vi "SignalObservation_NB.vi"(6 "error in (no error)":errorcluster, 8 "PllCharz Divider":string(combo)="Div1", 9 "Signal":string(combo)="VCO") -> (0 "error out":errorcluster)   [LabVIEW 2011]
doc: "This VI outputs a selected signal from the NB PLL.\n\nInputs:\n1. Signal: PLL Clock to output (Refclk, VCO, etc.).\n2. PllCharz Divider: Setting of the PllCharz divider (Div1 or Div16)."
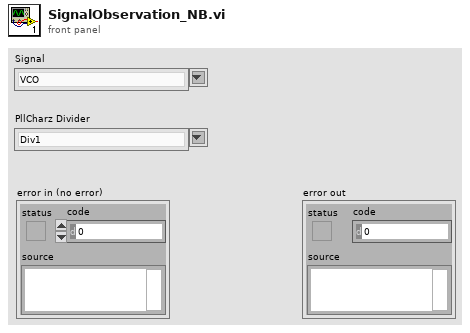
[diagram p1: front panel]
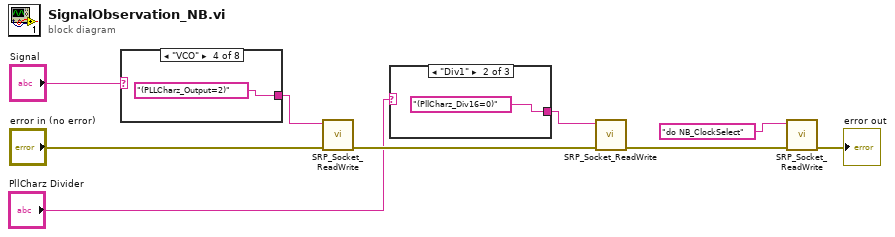
[diagram p0: block diagram]
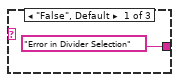
[diagram p2: hidden frame]
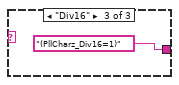
[diagram p3: hidden frame]
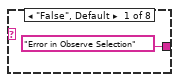
[diagram p4: hidden frame]
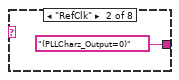
[diagram p5: hidden frame]
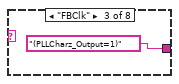
[diagram p6: hidden frame]
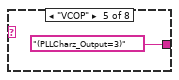
[diagram p7: hidden frame]
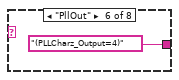
[diagram p8: hidden frame]
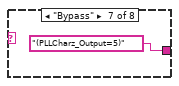
[diagram p9: hidden frame]
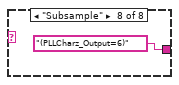
[diagram p10: hidden frame]
diagram:
  n1 = case shown="\"VCO\"" "Signal" {
    tunnel: ["Error in Observe Selection" "(PLLCharz_Output=0)" "(PLLCharz_Output=1)" "(PLLCharz_Output=2)" "(PLLCharz_Output=3)" "(PLLCharz_Output=4)" "(PLLCharz_Output=5)" "(PLLCharz_Output=6)"] -> w5
    frame "False", Default {
    }
    frame "RefClk" {
    }
    frame "FBClk" {
    }
    frame "VCO" {
    }
    frame "VCOP" {
    }
    frame "PllOut" {
    }
    frame "Bypass" {
    }
    frame "Subsample" {
    }
  }
  n2 = call "SRP_Socket_ReadWrite.vi"("error in (no error)"="error in (no error)", "Data In"=w5) -> ("error out"=w7:errorcluster)  [unwired: 7 in, 1 out]
  n3 = case shown="\"Div1\"" "PllCharz Divider" {
    tunnel: ["Error in Divider Selection" "(PllCharz_Div16=0)" "(PllCharz_Div16=1)"] -> w4
    frame "False", Default {
    }
    frame "Div1" {
    }
    frame "Div16" {
    }
  }
  n4 = call "SRP_Socket_ReadWrite.vi"("error in (no error)"=w7, "Data In"=w4) -> ("error out"=w6:errorcluster)  [unwired: 7 in, 1 out]
  n5 = call "SRP_Socket_ReadWrite.vi"("error in (no error)"=w6, "Data In"="do NB_ClockSelect") -> ("error out"=→"error out":errorcluster)  [unwired: 7 in, 1 out]
